vi "niDTS WLAN OFDM Tx Test Set Parameters.vi"(0 "Dummy Test Handle in":T9, 7 "Parameters":T1={"OFDM Data Rate (Mbps)"=enum."18", "Chains"=[TRUE, FALSE, FALSE, FALSE], "Bandwidth (Hz)"=enum."20 MHz", "Channel"=0, "Dut Tx Power (dBm)"=0.0, "16 symbols"=TRUE, "Payload Length (bytes)"=1, "Idle Interval (s)"=0.0, "External Attenuation (dB)"=[0.0, 0.0, 0.0, 0.0], "Acquisition "={"Acquisition Length Mode"=enum."AUTO", "Acquisition Length (s)"=3.0, "Auto Level"=FALSE}, "TXP Measurement"={"TXP Power Enable"=FALSE, "TXP Averages"=3}, "ModAcc Measurement"={"ModAcc Enable"=FALSE, "Header Detection"=enum."FIRST", "Averages"=3, "CFO Estimation"=enum."PAMBLE", "Amplitude Tracking"=FALSE, "Channel Tracking"=FALSE, "Time Tracking"=FALSE, "Phase Tracking"=enum."NONE", "Clock Offset Est"=FALSE, "Impairments Est"=FALSE}, "SEM Measurement"={"SEM Enable"=FALSE, "SEM Averages"=3, "Auto Span Enable"=FALSE, "Frequency Span (Hz)"=0.0, "Measurement Type"=enum."Standard", "Mask Frequencies (Hz)"=[], "Mask Power Offsets (dB)"=[]}, "OBW Measurement"={"OBW Enable"=FALSE, "OBW Averages"=3}} {"Acquisition"."Acquisition Length (s)" format="%#_6p"; "SEM Measurement"."Frequency Span (Hz)" format="%#_6p"; "Idle Interval (s)" format="%_3p"}, 11 "error in (no error)":errorcluster) -> (4 "Dummy Test Handle out":T9, 15 "error out":errorcluster)   [LabVIEW 2014, in "niDTS WLAN.lvlib"]
uses:
  niDTS WLAN.lvlib
  Tx Test/Includes/niDTS WLAN Tx Test INC Handle.ctl
  Tx Test/Objects/BASE_class/niDTS WLAN Tx Test.lvclass
  Includes/niDTS WLAN OFDM Tx Test INC Parameters.ctl
  Includes/niDTS WLAN INC OFDM Data Rate.ctl
  Includes/niDTS WLAN INC CH BW DSSS.ctl
  Includes/niDTS WLAN DUT INC Acquisition Parameters.ctl
  Includes/niDTS WLAN INC TXP Measurement Parameters.ctl
  Includes/niDTS WLAN OFDM Tx Test INC ModAcc Measurement Parameters.ctl
  Includes/niDTS WLAN INC SEM Measurement Parameters.ctl
  Includes/niDTS WLAN INC OBW Measurement Parameters.ctl
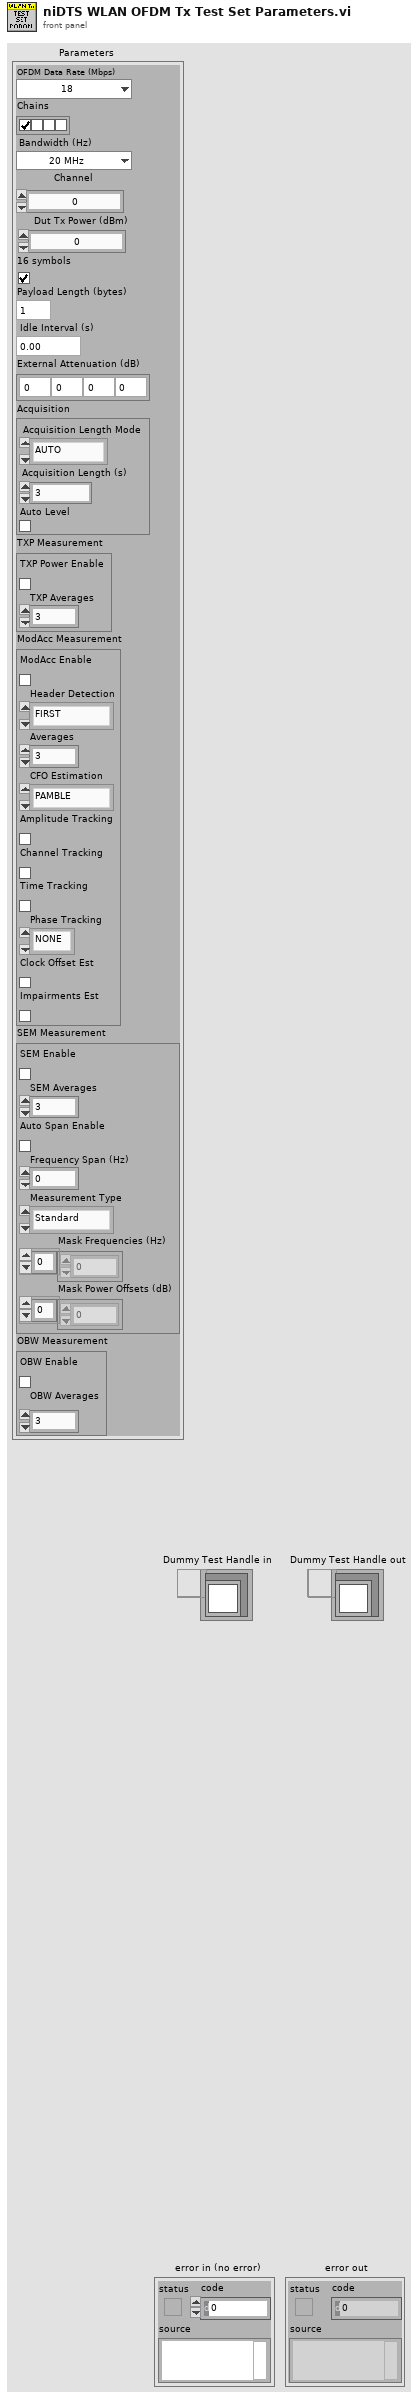
[diagram p1: front panel]
types:
  T1 = typedef "niDTS WLAN.lvlib/niDTS WLAN OFDM Tx Test INC Parameters.ctl" = cluster{"OFDM Data Rate (Mbps)":T2, "Chains":bool[], "Bandwidth (Hz)":T3, "Channel":i32, "Dut Tx Power (dBm)":dbl, "16 symbols":bool, "Payload Length (bytes)":i32, "Idle Interval (s)":dbl, "External Attenuation (dB)":dbl[], "Acquisition ":T4, "TXP Measurement":T5, "ModAcc Measurement":T6, "SEM Measurement":T7, "OBW Measurement":T8}
  T2 = typedef "niDTS WLAN.lvlib/niDTS WLAN INC OFDM Data Rate.ctl" = enum16{"6", "9", "12", "18", "24", "36", "48", "54"}
  T3 = typedef "niDTS WLAN.lvlib/niDTS WLAN INC CH BW DSSS.ctl" = enum16{"20 MHz"}
  T4 = typedef "niDTS WLAN.lvlib/niDTS WLAN DUT INC Acquisition Parameters.ctl" = cluster{"Acquisition Length Mode":enum16{"AUTO", "MANUAL"}, "Acquisition Length (s)":dbl, "Auto Level":bool}
  T5 = typedef "niDTS WLAN.lvlib/niDTS WLAN INC TXP Measurement Parameters.ctl" = cluster{"TXP Power Enable":bool, "TXP Averages":i32}
  T6 = typedef "niDTS WLAN.lvlib/niDTS WLAN OFDM Tx Test INC ModAcc Measurement Parameters.ctl" = cluster{"ModAcc Enable":bool, "Header Detection":enum16{"MANUAL", "FIRST", "ALL"}, "Averages":i32, "CFO Estimation":enum16{"PAMBLE", "PDATA"}, "Amplitude Tracking":bool, "Channel Tracking":bool, "Time Tracking":bool, "Phase Tracking":enum16{"NONE", "STANDARD", "CSF", "INSTANT"}, "Clock Offset Est":bool, "Impairments Est":bool}
  T7 = typedef "niDTS WLAN.lvlib/niDTS WLAN INC SEM Measurement Parameters.ctl" = cluster{"SEM Enable":bool, "SEM Averages":i32, "Auto Span Enable":bool, "Frequency Span (Hz)":dbl, "Measurement Type":enum16{"Standard", "Legacy", "Custom"}, "Mask Frequencies (Hz)":dbl[], "Mask Power Offsets (dB)":dbl[]}
  T8 = typedef "niDTS WLAN.lvlib/niDTS WLAN INC OBW Measurement Parameters.ctl" = cluster{"OBW Enable":bool, "OBW Averages":i32}
  T9 = typedef "niDTS WLAN.lvlib/niDTS WLAN Tx Test INC Handle.ctl" = refnum<data-value>
  T10 = typedef "niDTS WLAN.lvlib/niDTS WLAN Tx Test INC Parameters.ctl" = cluster{"Standard":T11, "DSSS Data Rate (Mbps)":T12, "OFDM Data Rate (Mbps)":T2, "MCS Index":i32, "N spatial streams":i32, "Chains":bool[], "BandWidth (Hz)":T13, "Channel":i32, "Gard Interval":T14, "FEC Coding":T15, "Dut Tx Power":dbl, "16 symbols":bool, "payload length bytes":i32, "idle interval":dbl, "External Attenuation":dbl[], "Acquisition Parameters ":T4, "TXP Measurement Parameters":T5, "ModAcc Measurement Paramaters":T16, "ModAcc DSSS Paramaters":T17, "SEM Measurement Parameters":T7, "OBW Measurement Parameters":T8, "DSSS Power Ramp":T19, "Enable Traces":bool}
  T11 = typedef "niDTS WLAN.lvlib/niDTS WLAN INC Standard.ctl" = enum16{"802.11 b DSSS", "802.11 a/g OFDM", "802.11 n HT", "802.11 ac VHT"}
  T12 = typedef "niDTS WLAN.lvlib/niDTS WLAN INC DSSS Data Rate.ctl" = enum16{"1", "2", "5.5", "11"}
  T13 = typedef "niDTS WLAN.lvlib/niDTS WLAN INC CH BW.ctl" = enum16{"20 MHz", "40 MHz", "80 MHz", "160 MHz"}
  T14 = typedef "niDTS WLAN.lvlib/niDTS WLAN INC GI.ctl" = enum16{"LONG", "SHORT"}
  T15 = typedef "niDTS WLAN.lvlib/niDTS WLAN INC FEC Coding.ctl" = enum16{"BCC", "LDPC"}
  T16 = typedef "niDTS WLAN.lvlib/niDTS WLAN INC ModAcc Measurement Parameters.ctl" = cluster{"ModAcc Enable":bool, "Header Detection":enum16{"MANUAL", "FIRST", "ALL"}, "Averages":i32, "Amplitude Tracking":bool, "Channel Tracking":bool, "Time Tracking":bool, "Phase Tracking":enum16{"NONE", "STANDARD", "CSF", "INSTANT"}, "Clock Offset Est":bool, "Impairments Est":bool, "CFO Estimation":enum16{"PAMBLE", "PDATA"}}
  T17 = typedef "niDTS WLAN.lvlib/niDTS WLAN INC DSSS ModAcc Measurement Parameters.ctl" = cluster{"DC Offset Compensation":bool, "Equalization":bool, "Phase Tracking":bool, "Chip Start Location":i16, "Max Chips Used":i16, "Pulse Shaping FilterType":T18, "Pulse Shaping Filter Coefficient":dbl}
  T18 = typedef "niDTS WLAN.lvlib/niDTS WLAN INC Pulse Shaping Filter Type.ctl" = enum16{"NONE", "RCOSINE", "RRCOSINE", "GAUSSIAN"}
  T19 = typedef "niDTS WLAN.lvlib/niDTS WLAN INC DSSS Power Ramp Parameters.ctl" = cluster{"Power Ramp Enable":bool, "Averages":i32, "Thresholds":cluster{"Up Low (%)":dbl, "Down Low (%)":dbl, "Up High (%)":dbl, "Down High (%)":dbl}}
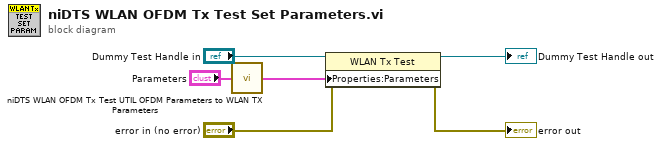
[diagram p0: block diagram]
diagram:
  n1 = call "niDTS WLAN OFDM Tx Test UTIL OFDM Parameters to WLAN TX Parameters.vi"("OFDM Parameters"="Parameters") -> ("WLAN Tx Parameters"=w1:T10)  [unwired: 14 in]
  n2 = property class="WLAN Tx Test"(reference="Dummy Test Handle in", error in="error in (no error)", "Properties:Parameters"=w1) -> (reference out=→"Dummy Test Handle out":T9, error out=→"error out":errorcluster)
